vi "GetDisplayName.vi"(8 "No Error":errorcluster, 11 "Display ID":T1) -> (0 "Error Out":errorcluster, 3 "Display Name":string)   [LabVIEW 2026, in "SDL3.lvlib" / "Video.lvlib"]
doc: "<B>Summary</B>\nGet the name of a display in UTF-8 encoding."
uses:
  Video.lvlib
  DisplayID--integer.ctl
  Stdinc/Strlen.vi
  Stdinc/Strlen.vi/c3f57b18-2899-4d18-8de7-ed42e0d99649.vi
  <vilib>/Utility/error.llb/Error Cluster From Error Code.vi
  Error/Error.lvlib
  LV-Utilities/LV-Utilities.lvlib
  Lib/SDL3.dll
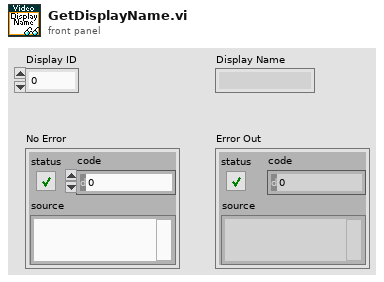
[diagram p1: front panel]
types:
  T1 = typedef "SDL3.lvlib/Video.lvlib/DisplayID--integer.ctl" = u32
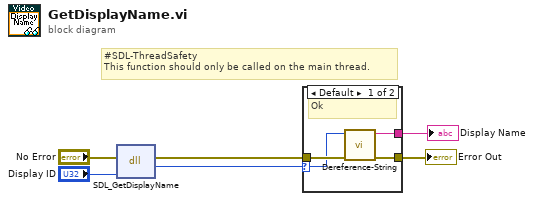
[diagram p0: block diagram]
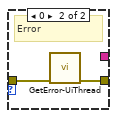
[diagram p2: hidden frame]
diagram:
  # "#SDL-ThreadSafety\nThis function should only be called on the main thread."
  n1 = dll-call lib="C:/Users/saukko/Dev/LV-SDL3/Sources/SDL3/Lib/SDL3.*" fn="SDL_GetDisplayName"(error in="No Error", "displayID"="Display ID") -> (error out=w4:errorcluster, "return type"=w2:i64)  [unwired: 3 in, 1 out]
  n2 = case shown="Default" w2 {
    selector: w2 -> [w8 _]
    tunnel: w4 -> [w10 w12]
    tunnel: [w9 w11] -> w5
    tunnel: [w7 _] -> w1
    frame Default {
      # "Ok"
      n3 = call "Dereference-String.vi"("No Error"=w10, "Str [const char *]"=w8) -> ("error out"=w9:errorcluster, "String"=w7:string)  [unwired: 8 in]
    }
    frame 0 {
      # "Error"
      n4 = call "GetError-UiThread.vi"("No Error"=w12) -> ("error out"=w11:errorcluster)  [unwired: 10 in]
    }
  }
  "Error Out" <- w5
  "Display Name" <- w1
